vi "Get Reader Status.vi"(8 "error in (no error)":errorcluster, 11 "Readable.lvclass in":refnum<class "Readable.lvclass">) -> (0 "error out":errorcluster, 2 "Status":string, 3 "Readable.lvclass out":refnum<class "Readable.lvclass">)   [LabVIEW 2009, in "Readable.lvclass"]
uses:
  Readable.lvclass
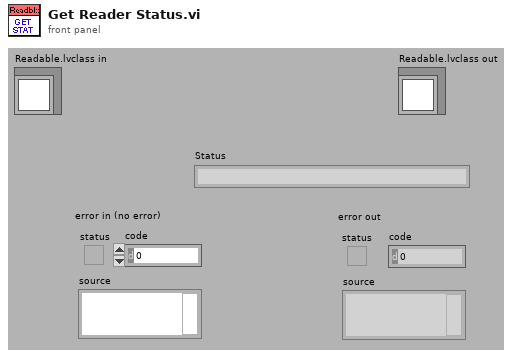
[diagram p1: front panel]
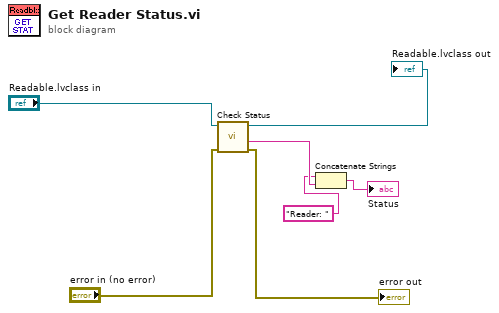
[diagram p0: block diagram]
diagram:
  n1 = call-dynamic "Check Status.vi"("error in (no error)"="error in (no error)", "Instrument in"="Readable.lvclass in") -> ("error out"=→"error out":errorcluster, "Status"=w2:string, "Instrument out"=→"Readable.lvclass out":refnum<class "Readable.lvclass">)  [unwired: 6 in, 1 out]
  n2 = Concatenate Strings("Reader: ", w2) -> (→"Status":string)
